vi "wavechart with adjustable domain.vi"() -> ()   [LabVIEW 2018]
panel:
  in  "Values to Display":dbl=100.0
  out "Waveform Chart":dynamicdata(graph)
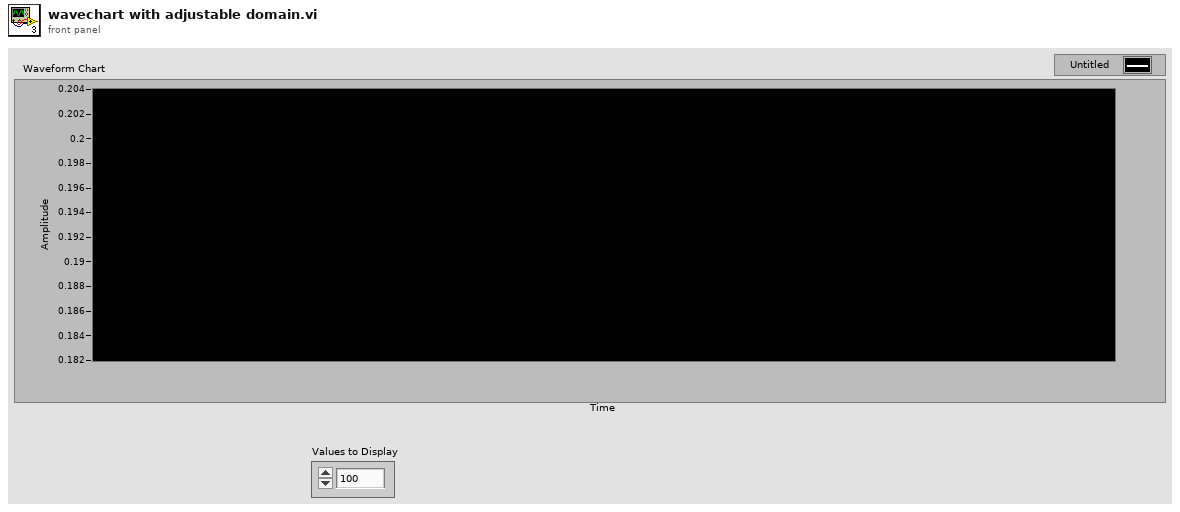
[diagram p1: front panel]
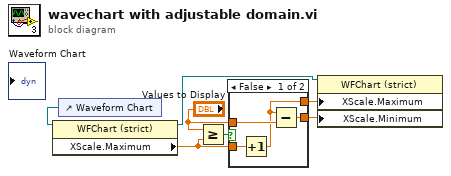
[diagram p0: block diagram]
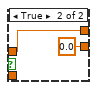
[diagram p2: hidden frame]
diagram:
  n1 = control-ref of="Waveform Chart"() -> (w7:refnum<vi>)
  n2 = property on="Property Node" class="WFChart (strict)"(reference=w7) -> (reference out=w1:refnum<vi>, "XScale.Maximum"=w2:dbl)  [unwired: 1 in, 1 out]
  n3 = Greater Or Equal?(x="Values to Display", y=w2) -> (x >= y?=w3:bool)
  n4 = case shown="False" w3 {
    tunnel: "Values to Display" -> [w9 w13]
    tunnel: w2 -> [w11 _]
    tunnel: [w8 w13] -> w5
    tunnel: [w10 0.0] -> w6
    frame False {
      n5 = Increment(x=w11) -> (x+1=w8:dbl)
      n6 = Subtract(x=w8, y=w9) -> (x-y=w10:dbl)
    }
    frame True {
    }
  }
  n7 = property on="Property Node" class="WFChart (strict)"(reference=w1, "XScale.Maximum"=w5, "XScale.Minimum"=w6) -> ()  [unwired: 1 in, 2 out]
